vi "_FPGA Write I32 Array.vi"(4 "error in":errorcluster, 5 "I32 Array":i32[](array[numeric]), 6 "Offset (0)":i32) -> (0 "error out":errorcluster, 2 "Next Offset":u16)   [LabVIEW 2012]
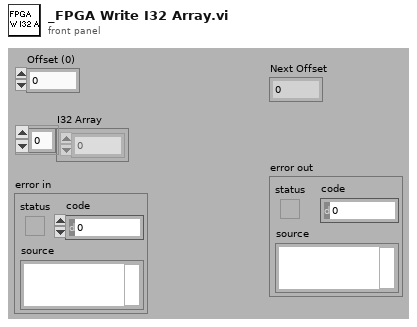
[diagram p1: front panel]
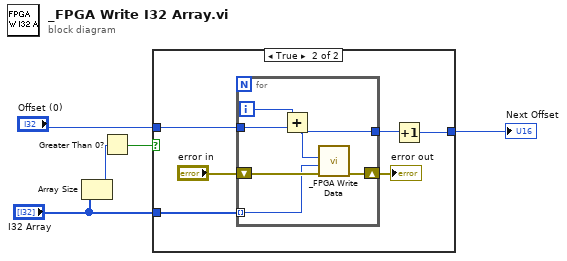
[diagram p0: block diagram]
diagram:
  n1 = Array Size(array="I32 Array") -> (size(s)=w2:i32)
  n2 = Greater Than 0?(x=w2) -> (x > 0?=w3:bool)
  n3 = case shown="True" w3 {
    tunnel: "Offset (0)" -> [w6 w12]
    tunnel: "I32 Array" -> [_ w11]
    tunnel: [w6 w7] -> w1
    frame False {
    }
    frame True {
      n4 = for {
        shift-right: [w17] -> w10
        shift-left: "error in" -> [w18]
        tunnel: w11 -> [w16] mode=indexing
        tunnel: w12 -> [w15]
        tunnel: [w14] -> w8
        i -> [w13]
        n5 = Add(x=w13, y=w15) -> (x+y=w14:i32)
        n6 = call "_FPGA Write Data.vi"("error in"=w18, "Data"=w16, "Address"=w14) -> ("error out"=w17:errorcluster)  [unwired: 3 in, 2 out]
      }
      "error out" <- w10
      n7 = Increment(x=w8) -> (x+1=w7:i32)
    }
  }
  "Next Offset" <- w1
